vi "ForceGraph3D.vi"(8 "number":dbl, 9 "Setpoint":dbl, 10 "k":dbl, 11 "Function":i32) -> (1 "force":dbl)   [LabVIEW 2023]
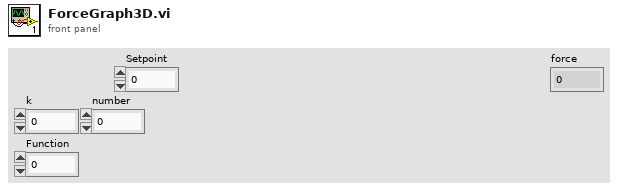
[diagram p1: front panel]
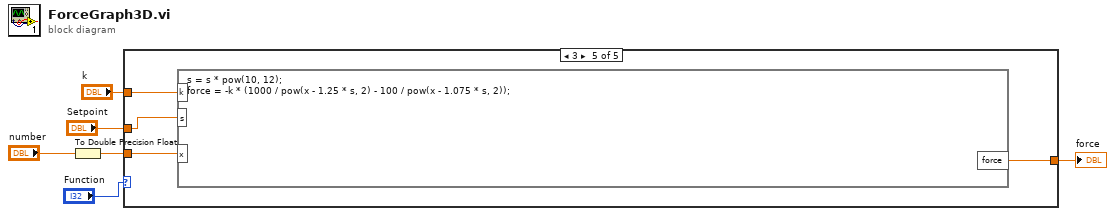
[diagram p0: block diagram]
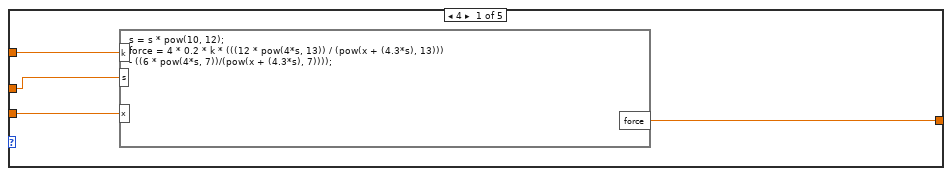
[diagram p2: hidden frame]
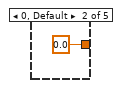
[diagram p3: hidden frame]
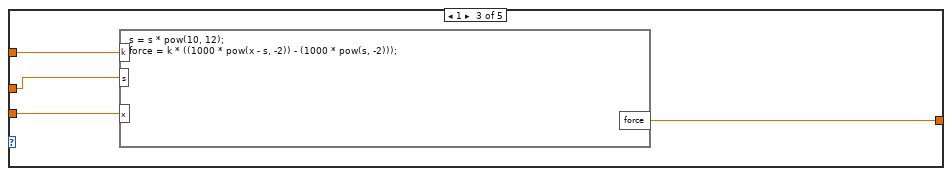
[diagram p4: hidden frame]
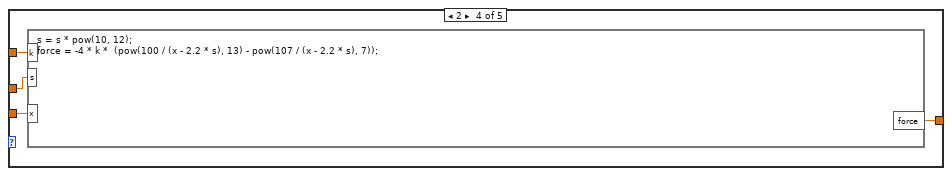
[diagram p5: hidden frame]
diagram:
  n1 = To Double Precision Float(number="number") -> (double precision float=w4:dbl)
  n2 = case shown="3" "Function" {
    tunnel: [w9 0.0 ("force") w15 w19 w20] -> w2
    tunnel: w4 -> [w10 _ w14 w18 w21]
    tunnel: "Setpoint" -> [w7 _ w13 w17 w22]
    tunnel: "k" -> [w8 _ w12 w16 w23]
    frame 4 {
      n3 = formula code="s = s * pow(10, 12);\nforce = 4 * 0.2 * k * (((12 * pow(4*s, 13)) / (pow(x + (4.3*s), 13))) \n- ((6 * pow(4*s, 7))/(pow(x + (4.3*s), 7))));"("x"=w10, "s"=w7, "k"=w8) -> ("force"=w9:dbl)
    }
    frame 0, Default {
    }
    frame 1 {
      n4 = formula code="s = s * pow(10, 12);\nforce = k * ((1000 * pow(x - s, -2)) - (1000 * pow(s, -2)));"("x"=w14, "s"=w13, "k"=w12) -> ("force"=w15:dbl)
    }
    frame 2 {
      n5 = formula code="s = s * pow(10, 12);\nforce = -4 * k *  (pow(100 / (x - 2.2 * s), 13) - pow(107 / (x - 2.2 * s), 7));"("x"=w18, "s"=w17, "k"=w16) -> ("force"=w19:dbl)
    }
    frame 3 {
      n6 = formula code="s = s * pow(10, 12);\nforce = -k * (1000 / pow(x - 1.25 * s, 2) - 100 / pow(x - 1.075 * s, 2));"("x"=w21, "s"=w22, "k"=w23) -> ("force"=w20:dbl)
    }
  }
  "force" <- w2
